vi "ep_Aggregate Harmonic.vi"(0 "complex spectra":T2(array[cluster]), 1 "restart (F)":bool, 7 "index":i32, 11 "error in (no error)":errorcluster) -> (4 "magnitude RMS":dbl[](array[numeric]), 6 "phase AVG":dbl[](array[numeric]), 14 "aggregated data valid?":bool, 15 "error out":errorcluster)   [LabVIEW 2012]
uses:
  <vilib>/addons/Electrical Power/PQ/Common/Controls/ep_AI Data Channel.ctl
  <vilib>/addons/Electrical Power/PQ/Common/Controls/ep_Aggregation Settings.ctl
  <vilib>/addons/Electrical Power/PQ/Common/Classes/System Info/EP System Info.lvclass
  <vilib>/addons/Electrical Power/PQ/Aggregation/Custom Aggregation (1D DBL Array).vi
  <vilib>/addons/Electrical Power/PQ/NI_EP_Power Quality.lvlib
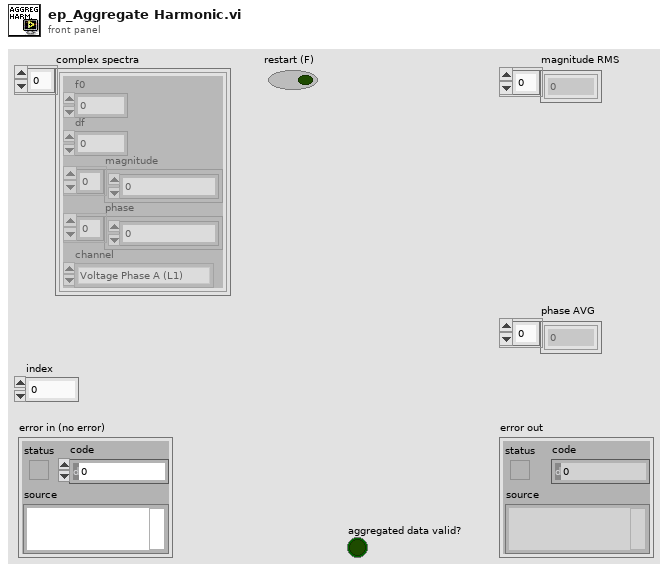
[diagram p1: front panel]
types:
  T1 = typedef "NI_EP_Power Quality.lvlib/ep_AI Data Channel.ctl" = enum16{"Voltage Phase A (L1)", "Voltage Phase B (L2)", "Voltage Phase C (L3)", "Voltage Phase N (Neutral)", "Current Phase A (L1)", "Current Phase B (L2)", "Current Phase C (L3)", "Current Phase N (Neutral)"}
  T2 = cluster{"f0":dbl, "df":dbl, "magnitude":dbl[], "phase":dbl[], "channel":T1}[]
  T3 = typedef "NI_EP_Power Quality.lvlib/ep_Aggregation Settings.ctl" = cluster{"interval":u32, "interval unit":enum16{"Runs", "Seconds", "Minutes", "Hours", "Days", "Weeks"}, "synchronization of intervals":enum16{"Not synchronized", "Interval rounded"}, "algorithm":enum16{"Average", "RMS"}}
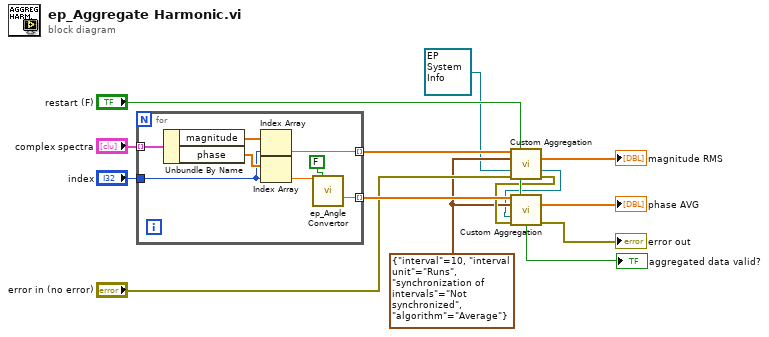
[diagram p0: block diagram]
diagram:
  w4 = T3 {"interval"=10, "interval unit"=enum."Runs", "synchronization of intervals"=enum."Not synchronized", "algorithm"=enum."Average"} ("aggregation settings")
  n1 = for {
    tunnel: "complex spectra" -> [w22] mode=indexing
    tunnel: [w19] -> w12 mode=indexing
    tunnel: [w15] -> w10 mode=indexing
    tunnel: "index" -> [w18]
    n2 = Unbundle By Name(w22) -> ("magnitude"=w21:dbl[], "phase"=w20:dbl[])
    n3 = Index Array(array=w21, index=w18) -> (element=w19:dbl)
    n4 = Index Array(array=w20, index=w18) -> (element=w17:dbl)
    n5 = call <vilib>:"ep_Angle Convertor.vi"("input angle"=w17, "input unit (F: radian)"=FALSE) -> ("angle in degrees (-180..180)"=w15:dbl)  [unwired: 10 in, 3 out]
  }
  n6 = call-poly <vilib>:"Custom Aggregation.vi"("data in"=w12, "reset? (F)"="restart (F)", "aggregation settings"=w4, "system info in"=refnum<class "EP System Info.lvclass"> refnum, "error in (no error)"="error in (no error)") -> ("aggregated averaged/RMS values"=→"magnitude RMS":dbl[], "system info out"=w3:refnum<class "EP System Info.lvclass">, "error out"=w6:errorcluster)  [unwired: 4 in, 4 out]
  n7 = call-poly <vilib>:"Custom Aggregation.vi"("data in"=w10, "reset? (F)"="restart (F)", "aggregation settings"=w4, "system info in"=w3, "error in (no error)"=w6) -> ("aggregated averaged/RMS values"=→"phase AVG":dbl[], "aggregated data valid?"=→"aggregated data valid?":bool, "error out"=→"error out":errorcluster)  [unwired: 4 in, 4 out]
